vi "Compresser OnOff.vi"(9 "Comp. Ref":string="My Compressor RefNum", 10 "Off":bool, 11 "On":bool) -> ()   [LabVIEW 2015, in "hhVI.lvlib"]
uses:
  <vilib>/Rock Robotics/WPI/Utilities/WPI_GetSetVariantRefNum.vi
  hhVI.lvlib
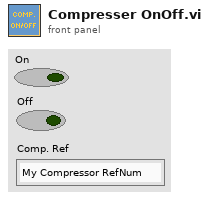
[diagram p1: front panel]
types:
  T1 = typedef "WPI_CompressorDevRef.ctl" = cluster{"DevStatus":errorcluster, "Pneumatics Control Module":u8}
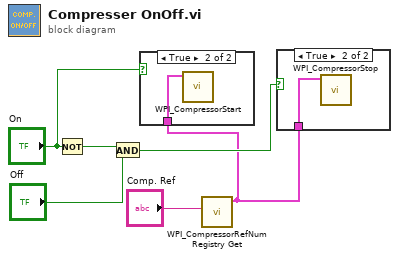
[diagram p0: block diagram]
diagram:
  n1 = Not(x="On") -> (.not. x?=w6:bool)
  n2 = And(x=w6, y="Off") -> (x .and. y?=w5:bool)
  n3 = call <vilib>:"WPI_CompressorRefNum Registry Get.vi"("refnum name"="Comp. Ref") -> ("CompressorDevRef"=w2:T1)  [unwired: 9 in, 1 out]
  n4 = case shown="True" "On" {
    tunnel: w2 -> [_ w7]
    frame False {
    }
    frame True {
      n5 = call <vilib>:"WPI_CompressorStart.vi"("CompressorDevRef"=w7) -> ()  [unwired: 9 in, 2 out]
    }
  }
  n6 = case shown="True" w5 {
    tunnel: w2 -> [_ w8]
    frame False {
    }
    frame True {
      n7 = call <vilib>:"WPI_CompressorStop.vi"("CompressorDevRef"=w8) -> ()  [unwired: 9 in, 2 out]
    }
  }
